vi "Get DI DAQ SMQ - polymorphic.vi"   [LabVIEW 2017, in "DAQ.lvclass"]
doc: "Developed by Kevin Thompson\nkevin@thompsonengineering.net\n\nCopyright 2018-2020\nThompson Engineering, LLC"
uses:
  DAQ.lvclass
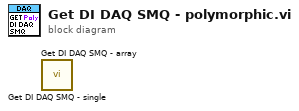
[diagram p0: block diagram]
diagram:
  n1 = call "Get DI DAQ SMQ - single.vi"() -> ()  [unwired: 9 in, 3 out]
  n2 = call "Get DI DAQ SMQ - array.vi"() -> ()  [unwired: 9 in, 3 out]
